vi "reg_check1.vi"() -> ()   [LabVIEW 2019]
uses:
  Inputs/Ctl/Parameter State short.ctl
  ctl/Y_state.ctl
  ctl/Z_State.ctl
  ctl/control param.ctl
  ctl/Y_short.ctl
  Y_switch_control.vi
  Y Limiter.vi
  PID Output Rate Limiter.vi
  PID Timing Estimation.vi
  control.lvlib
  Inputs/Inputs.lvlib
panel:
  in  "Start":bool
  out "End":bool
  out "T":u32
  out "Y 2":dbl format="%.2f"
  out "Y_State 2":T1={"Y_Source"=1, "Y_SetState"=5, "SP_Set"=0.0, "SP"=0.0, "PV"=0.0, "PV_State"={"code"=0, "visible"=FALSE, "color"=0}, "Y_preSet"=0.0, "Y_Set"=0.0, "Y"=0.0, "Y_State"={"code"=0, "visible"=FALSE, "color"=0}, "YB"=FALSE} {"Y" format="%.2f"; "Y_preSet" format="%.2f"; "SP" step=0.01 format="%.2f"; "Y_Set" format="%.2f"; "PV" step=0.01 format="%.2f"; "SP_Set" step=0.01 format="%.2f"}
  out "YB":bool
  in  "XB24 (F)":bool
  in  "control param":T3={"proportional gain (Kc)"=1.0, "integral time (Ti, s)"=10.0, "derivative time (Td, s)"=1.0, "output high"=100.0, "output high start"=40.0, "output high stop"=40.0, "alr value"=0.0, "output low"=0.0, "output rate (EGU/s)"=5.0, "setpoint max"=100.0, "setpoint rate (EGU/min)"=10.0, "stop rate (EGU/min)"=5.0} {"setpoint max" format="%.2f"; "stop rate (EGU/min)" min=0.001 format="%.2f"; "setpoint rate (EGU/min)" min=0.001 format="%.2f"; "output high stop" format="%.2f"; "output high start" format="%.2f"; "output rate (EGU/s)" min=0.001 format="%.2f"; "output low" format="%.2f"; "alr value" format="%.2f"; "output high" format="%.2f"; "derivative time (Td, s)" format="%.3f"; "integral time (Ti, s)" format="%.3f"; "proportional gain (Kc)" format="%.3f"}
  in  "Z":T4
  in  "controls Y":cluster{"Y_H":dbl, "Y_A":dbl, "Y_D":dbl} {"Y_H" format="%.2f"; "Y_D" format="%#_13g"; "Y_A" format="%#_13g"}
  in  "Y_Set":T6={"Y_HSw"=1, "Y_HSetState"=enum."auto", "Y_ASetState"=enum."auto", "Y_DSetState"=enum."auto"} {"Y_HSw" max=2 step=1}
  in  "Y_State":T2
  in  "Y":dbl step=0.01 format="%.2f"
  in  "PV_State":T2
  in  "PV":dbl step=0.01 format="%.2f"
  in  "SP":dbl caption="setpoint" step=0.01 format="%.2f"
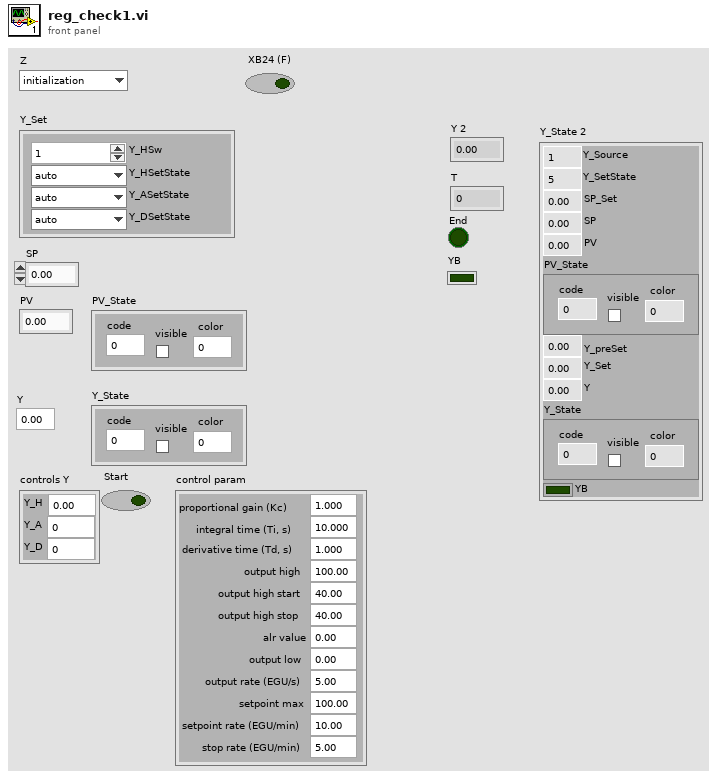
[diagram p1: front panel]
types:
  T1 = typedef "control.lvlib/Y_short.ctl" = cluster{"Y_Source":u8, "Y_SetState":u8, "SP_Set":dbl, "SP":dbl, "PV":dbl, "PV_State":T2, "Y_preSet":dbl, "Y_Set":dbl, "Y":dbl, "Y_State":T2, "YB":bool}
  T2 = typedef "Inputs.lvlib/Parameter State short.ctl" = cluster{"code":i32, "visible":bool, "color":u32}
  T3 = typedef "control.lvlib/control param.ctl" = cluster{"proportional gain (Kc)":dbl, "integral time (Ti, s)":dbl, "derivative time (Td, s)":dbl, "output high":dbl, "output high start":dbl, "output high stop":dbl, "alr value":dbl, "output low":dbl, "output rate (EGU/s)":dbl, "setpoint max":dbl, "setpoint rate (EGU/min)":dbl, "stop rate (EGU/min)":dbl}
  T4 = typedef "control.lvlib/Z_State.ctl" = enum8{"initialization", "alarm", "disabled", "not ready", "stop ready", "reserv", "switched off", "reserv2", "switched on", "check", "on min", "decrease out", "on", "increase out", "on max"}
  T5 = typedef "control.lvlib/Y_state.ctl" = enum8{"initialize", "alarm", "min", "stop", "hand", "auto", "max"}
  T6 = cluster{"Y_HSw":u32, "Y_HSetState":T5, "Y_ASetState":T5, "Y_DSetState":T5}
  T7 = typedef "control.lvlib/Y.ctl" = cluster{"Y_Source":T8, "Y_SetState":T5, "SP_Set":dbl, "SP":dbl, "PV":dbl, "PV_State":T2, "Y_preSet":dbl, "Y_Set":dbl, "Y":dbl, "Y_State":T2, "YB":bool}
  T8 = typedef "control.lvlib/Y_source.ctl" = enum8{"initialize", "local disabled", "local hand", "hand", "auto", "dist"}
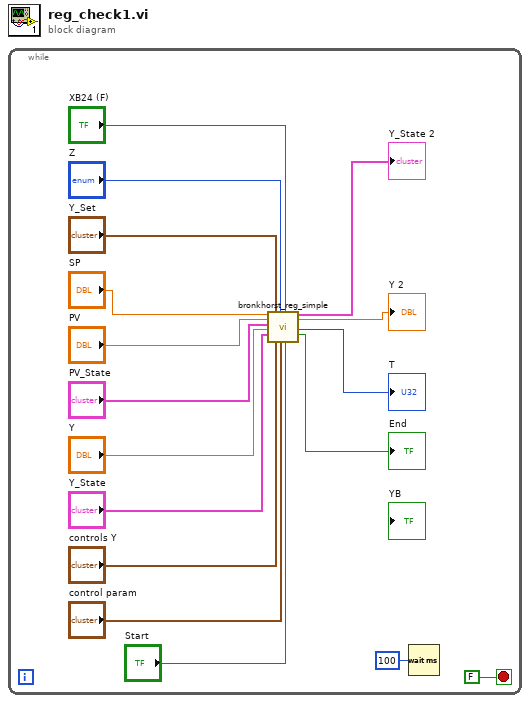
[diagram p0: block diagram]
diagram:
  n1 = while {
    stop <- FALSE stop-if-true
    n2 = call "bronkhorst_reg_simple.vi"("SP"="SP", "PV"="PV", "PV_State"="PV_State", "Y"="Y", "Y_State"="Y_State", "Y_Set"="Y_Set", "controls Y"="controls Y", "Z"="Z", "control param"="control param", "XB24 (F)"="XB24 (F)", "Start"="Start") -> ("Y_State"=→"Y_State 2":T7, "Y"=→"Y 2":dbl, "T"=→"T":u32, "End"=→"End":bool)  [unwired: 5 in]
    n3 = Wait (ms)(milliseconds to wait=u32 100) -> ()  [unwired: 1 out]
  }
